vi "calculate_p_hat_perpendicular.vi"(8 "Error In":errorcluster, 10 "xi":dbl, 11 "gamma":dbl) -> (0 "Error Out":errorcluster, 3 "p hat perpendicular":dbl[](array[numeric]))   [LabVIEW 2019]
doc: "Calculate phi from formula 4 in Wilen(2000). All inputs and outputs are in degrees."
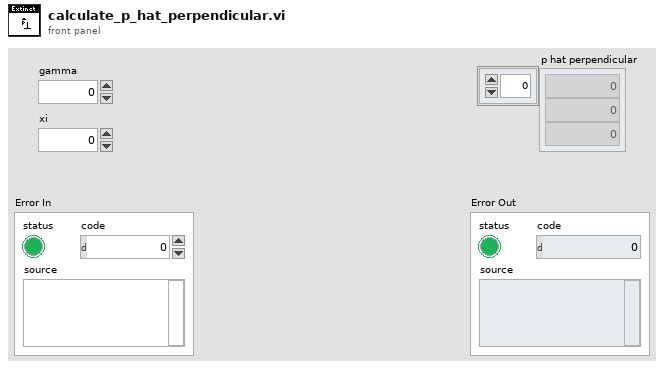
[diagram p1: front panel]
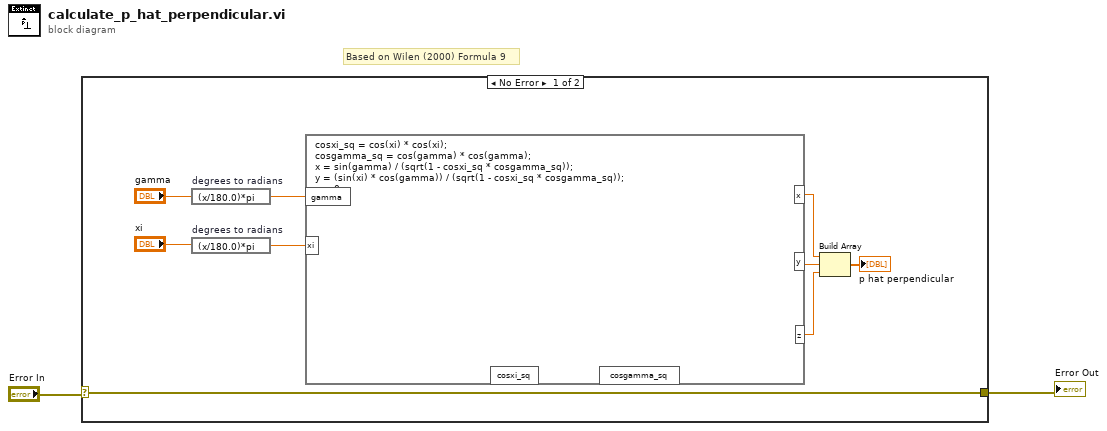
[diagram p0: block diagram]
diagram:
  # "Based on Wilen (2000) Formula 9"
  n1 = case shown="No Error" "Error In" {
    selector: "Error In" -> [w11 w12]
    tunnel: [w11 w12] -> w1
    frame No Error {
      n2 = expression code="(x/180.0)*pi" "degrees to radians"("gamma") -> (w10:dbl)
      n3 = expression code="(x/180.0)*pi" "degrees to radians"("xi") -> (w9:dbl)
      n4 = formula code="cosxi_sq = cos(xi) * cos(xi);\ncosgamma_sq = cos(gamma) * cos(gamma);\nx = sin(gamma) / (sqrt(1 - cosxi_sq * cosgamma_sq));\ny = (sin(xi) * cos(gamma)) / (sqrt(1 - cosxi_sq * cosgamma_sq));\nz = 0;"("gamma"=w10, "xi"=w9) -> ("x"=w5:dbl, "y"=w6:dbl, "z"=w4:dbl)  [unwired: 2 out]
      n5 = Build Array(w5, w6, w4) -> (→"p hat perpendicular":dbl[])
    }
    frame Error {
    }
  }
  "Error Out" <- w1
